vi "Entry Console View.vi"(8 "error in (no error)":errorcluster, 11 "View Model":T2) -> (0 "error out":errorcluster, 3 "View Model":T2)   [LabVIEW 2017]
doc: "The interface via wich the user selects the car wash options to be executed by the car wash controller."
uses:
  View Model/Controls/View Model.ctl
  View Model/Controls/Shared Model.ctl
  Error Handler/Controls/Error Model.ctl
  Error Handler/Controls/Error Data.ctl
  Error Handler/Controls/Error Level.ctl
  Configuration/Controls/Config Model.ctl
  Configuration/Controls/Config Record.ctl
  Configuration/Controls/Config Data.ctl
  Configuration/Controls/Config Command.ctl
  Controller/Controls/Controler Model.ctl
  Vehicle Position View/Controls/Vehicle - Station Slider.ctl
  Controller/Controls/Controller - Wash Step.ctl
  Controls/Entry Console - Wash Steps.ctl
panel:
  in  "Start Wash":bool
  in  "Wash Steps":T1
  # "Entry Console"
  # "[Covers: UI2]"
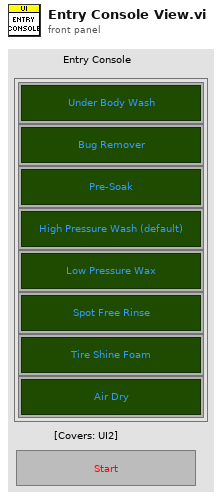
[diagram p1: front panel]
types:
  T1 = typedef "Entry Console - Wash Steps.ctl" = cluster{"Under Body Wash":bool, "Bug Remover":bool, "Pre-Soak":bool, "High Pressure Wash":bool, "Low Pressure Wax":bool, "Spot Free Rinse":bool, "Tire Shine Foam":bool, "Air Dry":bool}
  T2 = typedef "View Model.ctl" = cluster{"Shared Model":T3, "Error Model":T4, "Config Model":T5, "Controler Model":T6}
  T3 = typedef "Shared Model.ctl" = cluster{"Stop":refnum<user-event>, "Stop DVR":refnum<data-value>}
  T4 = typedef "Error Model.ctl" = cluster{"Error":refnum<user-event>}
  T5 = typedef "Config Model.ctl" = cluster{"Config Recs DVR":refnum<data-value>, "Config Data":refnum<user-event>, "Config Lock":refnum<user-event>, "Config Lock DVR":refnum<data-value>}
  T6 = typedef "Controler Model.ctl" = cluster{"Station":refnum<user-event>, "Wash Sequence":refnum<data-value>, "Wash Step Exec":refnum<user-event>, "Wash Step Start":refnum<user-event>, "Wash Step Complete":refnum<user-event>, "Wash Cycle Complete":refnum<user-event>, "Wash Cycle Start":refnum<user-event>}
  T7 = enum8{"Enabled", "Disabled", "Disabled and Grayed Out"}
  T8 = typedef "Controller - Wash Step.ctl" = enum16{"Under Body Wash", "Bug Remover", "Pre-Soak", "High Pressure Wash", "Low Pressure Wax", "Spot Free Rinse", "Tire Shine Foam", "Air Dry"}
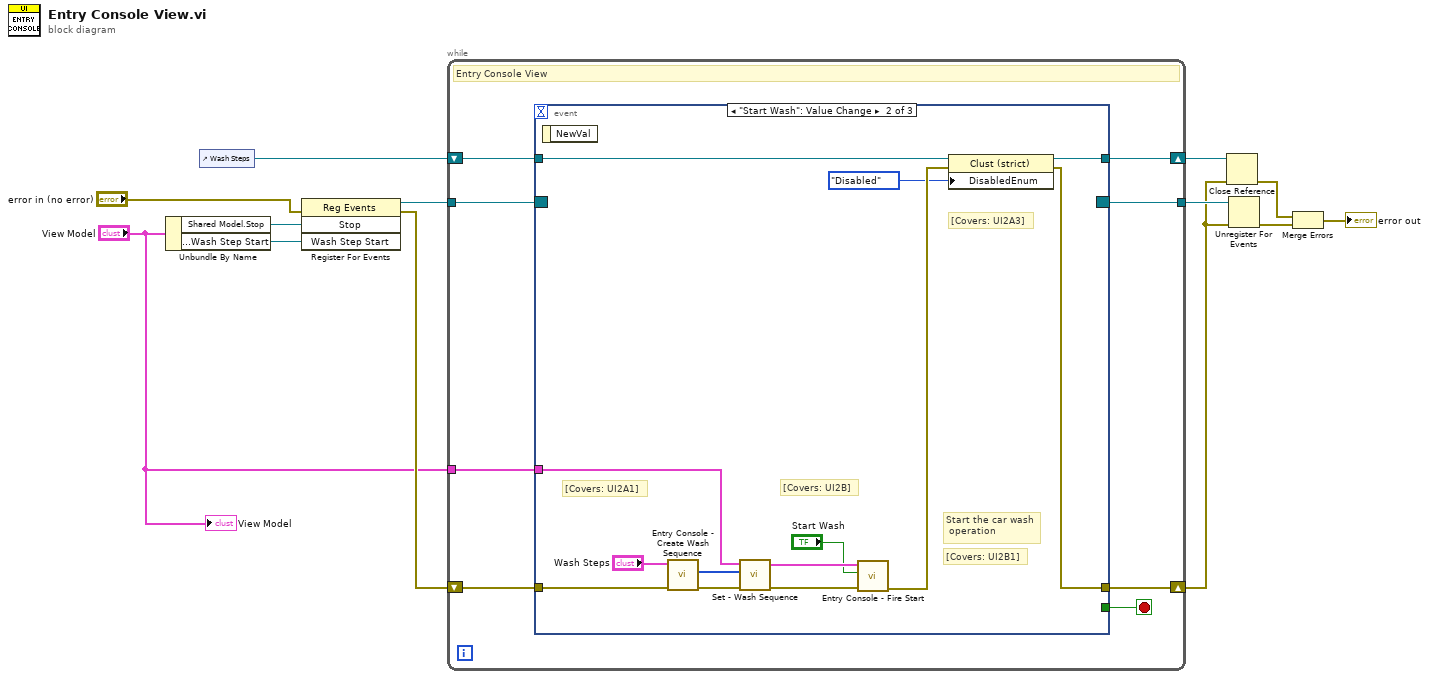
[diagram p0: block diagram]
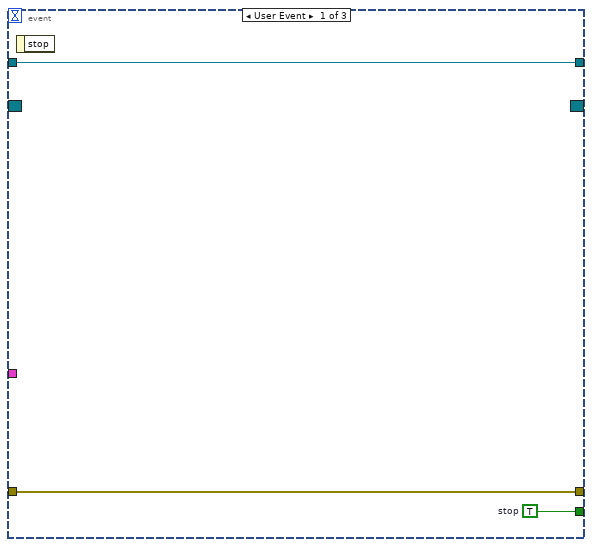
[diagram p2: hidden frame]
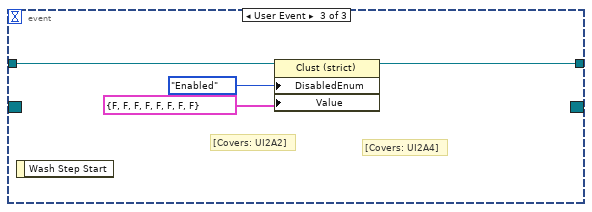
[diagram p3: hidden frame]
diagram:
  n1 = Unbundle By Name("View Model") -> ("Shared Model.Stop"=w13:refnum<user-event>, "Controler Model.Wash Step Start"=w6:refnum<user-event>)
  n2 = control-ref of="Wash Steps"() -> (w7:refnum<vi>)
  n3 = register-events(error in="error in (no error)", w13, w6) -> (reference out=w11:refnum<event-registration>, error out=w10:errorcluster)  [unwired: 1 in]
  n4 = while {
    tunnel: w11 -> [w21]
    shift-right: [w19] -> w4
    shift-left: w10 -> [w20]
    tunnel: [w17] -> w9
    tunnel: "View Model" -> [w16]
    shift-right: [w14] -> w5
    shift-left: w7 -> [w15]
    stop <- w18 stop-if-true
    # "Entry Console View"
    n5 = event shown="[1] \"Start Wash\": Value Change" {
      selector: w21 -> [_ _ _]
      dyn-events: [_ _ _] -> w17
      timeout: _ -> [_ _ _]
      tunnel: w20 -> [w24 w37 _]
      tunnel: [w24 w26 _] -> w19
      tunnel: [w23 _ _] -> w18
      tunnel: w16 -> [_ w34 _]
      tunnel: w15 -> [w22 w29 w41]
      tunnel: [w22 w28 w40] -> w14
      event User Event {
        w23 = TRUE  # stop
        n6 = event-data() -> ()  [unwired: 1 in, 1 out]
      }
      event "Start Wash": Value Change {
        # "[Covers: UI2B1]"
        # "Start the car wash\n operation"
        # "[Covers: UI2B]"
        # "[Covers: UI2A3]"
        # "[Covers: UI2A1]"
        n7 = event-data() -> ()  [unwired: 1 in, 1 out]
        n8 = call "Entry Console - Create Wash Sequence.vi"("error in (no error)"=w37, "Wash Steps"="Wash Steps") -> ("error out"=w36:errorcluster, "Wash Sequence"=w35:T8[])  [unwired: 8 in]
        n9 = call "Set - Wash Sequence.vi"("error in (no error)"=w36, "Wash Sequence"=w35, "View Model"=w34) -> ("error out"=w33:errorcluster, "View Model"=w32:T2)  [unwired: 7 in]
        n10 = call "Entry Console - Fire Start.vi"("error in (no error)"=w33, "Start"="Start Wash", "View Model"=w32) -> ("error out"=w27:errorcluster)  [unwired: 7 in, 1 out]
        n11 = property class="Clust (strict)"(reference=w29, error in=w27, "DisabledEnum"=T7."Disabled" ("Disabled")) -> (reference out=w28:refnum<vi>, error out=w26:errorcluster)
      }
      event User Event {
        # "[Covers: UI2A4]"
        # "[Covers: UI2A2]"
        n12 = event-data() -> ()  [unwired: 1 in, 1 out]
        n13 = property class="Clust (strict)"(reference=w41, "DisabledEnum"=T7."Enabled" ("Disabled"), "Value"=T1 {"Under Body Wash"=FALSE, "Bug Remover"=FALSE, "Pre-Soak"=FALSE, "High Pressure Wash"=FALSE, "Low Pressure Wax"=FALSE, "Spot Free Rinse"=FALSE, "Tire Shine Foam"=FALSE, "Air Dry"=FALSE}) -> (reference out=w40:refnum<vi>)  [unwired: 1 in, 1 out]
      }
    }
  }
  n14 = Close Reference(reference=w5, error in (no error)=w4) -> (error out=w2:errorcluster)
  n15 = Unregister For Events(event registration refnum=w9, error in=w4) -> (error out=w3:errorcluster)
  n16 = Merge Errors(w2, w3) -> (→"error out":errorcluster)
  "View Model" <- "View Model"
